vi "Ak_Array.vi"(9 "Ak 30min":dbl, 10 "Ak_axis":i32) -> (3 "Ak Aray":dbl[](array[numeric]))   [LabVIEW 2019]
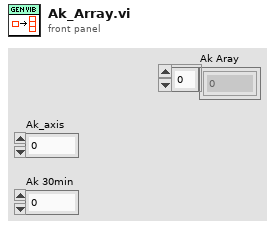
[diagram p1: front panel]
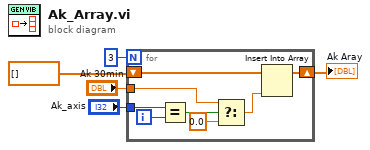
[diagram p0: block diagram]
diagram:
  n1 = for {
    N: 3 -> [_]
    tunnel: "Ak_axis" -> [w12]
    tunnel: "Ak 30min" -> [w10]
    shift-right: [w7] -> w3
    shift-left: dbl[] [] -> [w6]
    i -> [w13]
    n2 = Equal?(x=w12, y=w13) -> (x = y?=w11:bool)
    n3 = Select(t=w10, s=w11, f=0.0) -> (s? t:f=w8:dbl)
    n4 = Insert Into Array(array=w6, new element=w8) -> (w7:dbl[])  [unwired: 1 in]
  }
  "Ak Aray" <- w3
